vi "Main Page.vi"(8 "error in":errorcluster, 11 "Node Ptr":T1 format="%.0x") -> (0 "error out":errorcluster)   [LabVIEW 2026, in "SystemMonitor System Explorer.lvlib"]
uses:
  <vilib>/NI VeriStand/Custom Device API/Custom Device Item Ref.ctl
  <vilib>/NI VeriStand/Custom Device API/Get Item Property (U16).vi
  <vilib>/NI VeriStand/Custom Device API/Set Item Property (U16).vi
  SystemMonitor System Explorer.lvlib
  <vilib>/NI VeriStand/Custom Device API/Custom Device API.lvlib
  C:/Program Files/National Instruments/VeriStand 2026/NationalInstruments.VeriStand.Controls.dll
  Program Files/National Instruments/VeriStand 2026/NationalInstruments.VeriStand.Controls.dll
panel:
  in  "Timeout":u16 caption="Async Timeout (ms)"
  in  "PagePropertyEditor":refnum<k24>(container)
  out "Version":string
  in  "Browser":refnum<k7>(container)
  in  "General Header":cluster{"Section Name":string}={"Section Name"="General Custom Device Settings"}
  in  "Description":string
  in  "Name":string
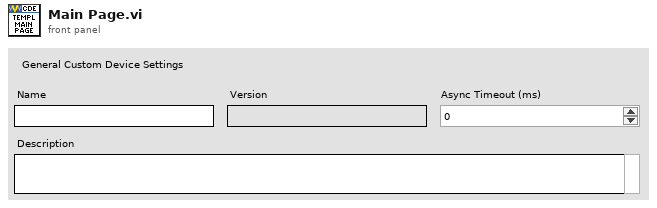
[diagram p1: front panel]
types:
  T1 = typedef "Custom Device API.lvlib/Custom Device Item Ref.ctl" = u64
  T2 = typedef "Custom Device API.lvlib/Custom Device Item Info.ctl" = cluster{"Name":string, "Is Channel":bool, "GUID":string, "Is Waveform":bool}
  T3 = typedef "Custom Device API.lvlib/Custom Device Commands.ctl" = enum16{"Default", "Item renamed", "Shutdown", "Dynamic button pressed"}
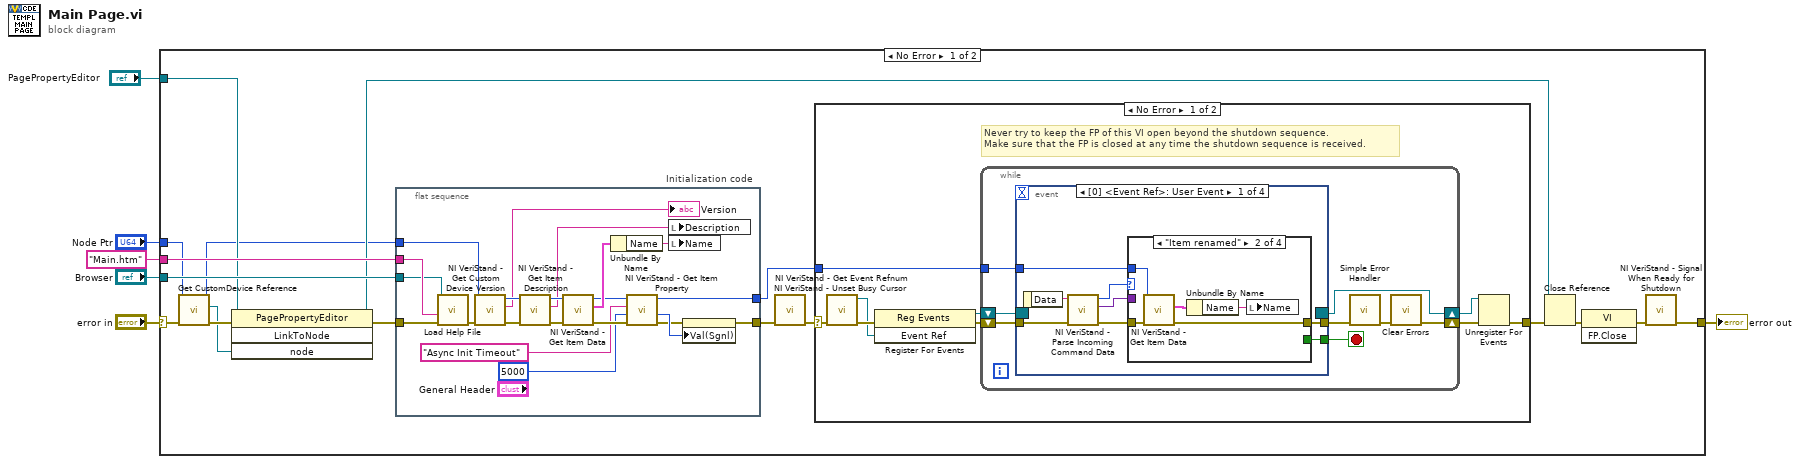
[diagram p0: block diagram]
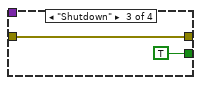
[diagram p3: hidden frame]
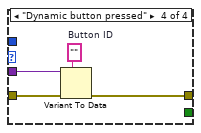
[diagram p4: hidden frame]
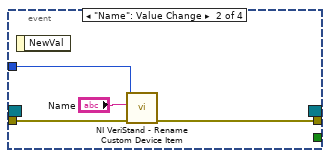
[diagram p5: hidden frame]
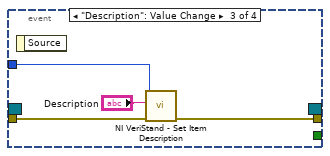
[diagram p6: hidden frame]
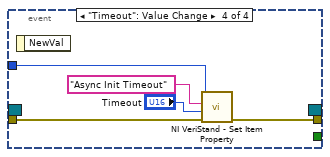
[diagram p7: hidden frame]
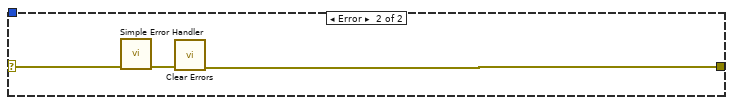
[diagram p8: hidden frame]
diagram:
  n1 = case shown="No Error" "error in" {
    selector: "error in" -> [w16 w98]
    tunnel: [w23 w98] -> w2
    tunnel: "Node Ptr" -> [w7 _]
    tunnel: "Browser" -> [w22 _]
    tunnel: "Main.htm" ("HTML File") -> [w21 _]
    tunnel: "PagePropertyEditor" -> [w9 _]
    frame No Error {
      n2 = call "Get CustomDevice Reference.vi"("error in"=w16, "Node Ptr"=w7) -> ("error out"=w12:errorcluster, "Custom Device"=w11:refnum<k24>, "Node Ptr"=w8:T1)  [unwired: 7 in]
      n3 = invoke class="PagePropertyEditor" method="LinkToNode"(reference=w9, error in=w12, "node"=w11) -> (reference out=w10:refnum<k24>, error out=w15:errorcluster)  [unwired: 1 in, 2 out]
      n4 = flat-sequence "Initialization code" {
        tunnel: w15 -> [w42]
        tunnel: w8 -> [w38]
        tunnel: [w24] -> w17
        tunnel: [w30] -> w18
        tunnel: w22 -> [w32]
        tunnel: w21 -> [w33]
        frame #0 {
          n5 = call "Load Help File.vi"("error in"=w42, "HTML File to Load"=w33, "Browser"=w32) -> ("error out"=w41:errorcluster)  [unwired: 8 in]
          n6 = call <vilib>:"NI VeriStand - Get Custom Device Version.vi"("error in (no error)"=w41, "Device Ref in"=w38) -> ("error out"=w43:errorcluster, "Value"=→"Version":string, "Device Ref out"=w37:T1)  [unwired: 7 in]
          n7 = call <vilib>:"NI VeriStand - Get Item Description.vi"("error in (no error)"=w43, "Item Ref in"=w37) -> ("error out"=w44:errorcluster, "Description"=w34:string, "Item Ref out"=w40:T1)  [unwired: 7 out]
          n8 = call <vilib>:"NI VeriStand - Get Item Data.vi"("error in (no error)"=w44, "Item Ref in"=w40) -> ("error out"=w29:errorcluster, "Item Info"=w39:T2, "Item Ref out"=w31:T1)  [unwired: 7 out]
          n9 = Unbundle By Name(w39) -> ("Name"=w35:string)
          n10 = call-poly <vilib>:"NI VeriStand - Get Item Property.vi"("error in (no error)"=w29, "Default Value"=u16 5000, "Property Name"="Async Init Timeout", "Item Ref in"=w31) -> ("error out"=w25:errorcluster, "Value"=w26:u16, "Item Ref out"=w30:T1)  [unwired: 4 in, 1 out]
          n11 = local write "Description"(w34) -> ()
          n12 = local write "Name"(w35) -> ()
          n13 = property on="Timeout" class="DigNum (strict)"(error in=w25, "Val(Sgnl)"=w26) -> (error out=w24:errorcluster)  [unwired: 1 in, 1 out]
        }
      }
      n14 = call <vilib>:"NI VeriStand - Unset Busy Cursor.vi"("error in (no error)"=w17) -> ("error out"=w19:errorcluster)  [unwired: 10 out]
      n15 = case shown="No Error" w19 {
        selector: w19 -> [w49 w97]
        tunnel: [w51 w95] -> w14
        tunnel: w18 -> [w45 _]
        frame No Error {
          # "Never try to keep the FP of this VI open beyond the shutdown sequence.\nMake sure that the FP is closed at any time the shutdown sequence is received."
          n16 = call <vilib>:"NI VeriStand - Get Event Refnum.vi"("error in (no error)"=w49) -> ("error out"=w53:errorcluster, "Event Ref"=w47:refnum<user-event>)  [unwired: 9 out]
          n17 = register-events(error in=w53, w47) -> (reference out=w46:refnum<event-registration>, error out=w50:errorcluster)  [unwired: 1 in]
          n18 = while {
            tunnel: w45 -> [w54]
            shift-right: [w58] -> w52
            shift-left: w50 -> [w61]
            shift-right: [w57] -> w48
            shift-left: w46 -> [w56]
            stop <- w55 stop-if-true
            n19 = event shown="[0] <Event Ref>: User Event" {
              selector: w56 -> [_ _ _ _]
              dyn-events: [_ _ _ _] -> w57
              timeout: _ -> [_ _ _ _]
              tunnel: w61 -> [w69 w85 w89 w94]
              tunnel: [w64 _ _ _] -> w55
              tunnel: [w67 w84 w88 w93] -> w60
              tunnel: w54 -> [w63 w83 w87 w91]
              event User Event {
                n20 = event-data() -> ("Data"=w66:string)  [unwired: 1 out]
                n21 = call <vilib>:"NI VeriStand - Parse Incoming Command Data.vi"("error in (no error)"=w69, "Incoming data"=w66) -> ("error out"=w68:errorcluster, "Outgoing data"=w62:variant, "Action"=w65:T3)  [unwired: 7 out]
                n22 = case shown="\"Item renamed\"" w65 {
                  tunnel: w68 -> [w70 w75 w77 w81]
                  tunnel: [_ _ TRUE _] -> w64
                  tunnel: [w70 w74 w77 w80] -> w67
                  tunnel: w63 -> [_ w73 _ _]
                  tunnel: w62 -> [_ _ _ w79]
                  frame "Default", Default {
                  }
                  frame "Item renamed" {
                    n23 = call <vilib>:"NI VeriStand - Get Item Data.vi"("error in (no error)"=w75, "Item Ref in"=w73) -> ("error out"=w74:errorcluster, "Item Info"=w72:T2)  [unwired: 8 out]
                    n24 = Unbundle By Name(w72) -> ("Name"=w71:string)
                    n25 = local write "Name"(w71) -> ()
                  }
                  frame "Shutdown" {
                  }
                  frame "Dynamic button pressed" {
                    w78 = ""  # Button ID
                    n26 = Variant To Data(error in=w81, type=w78, Variant=w79) -> (error out=w80:errorcluster)  [unwired: 1 out]
                  }
                }
              }
              event "Name": Value Change {
                n27 = event-data() -> ()  [unwired: 2 out]
                n28 = call <vilib>:"NI VeriStand - Rename Custom Device Item.vi"("error in (no error)"=w85, "New Name"="Name", "Item Ref in"=w83) -> ("error out"=w84:errorcluster)  [unwired: 1 in, 7 out]
              }
              event "Description": Value Change {
                n29 = event-data() -> ()  [unwired: 2 out]
                n30 = call <vilib>:"NI VeriStand - Set Item Description.vi"("error in (no error)"=w89, "Description"="Description", "Item Ref in"=w87) -> ("error out"=w88:errorcluster)  [unwired: 8 out]
              }
              event "Timeout": Value Change {
                n31 = event-data() -> ()  [unwired: 2 out]
                n32 = call-poly <vilib>:"NI VeriStand - Set Item Property.vi"("error in (no error)"=w94, "Value"="Timeout", "Property Name"="Async Init Timeout", "Item Ref in"=w91) -> ("error out"=w93:errorcluster)  [unwired: 5 in, 2 out]
              }
            }
            n33 = call <vilib>:"Simple Error Handler.vi"("error in (no error)"=w60) -> ("error out"=w59:errorcluster)  [unwired: 1 in, 7 out]
            n34 = call <vilib>:"Clear Errors.vi"("error in (no error)"=w59) -> ("error out"=w58:errorcluster)  [unwired: 1 in, 5 out]
          }
          n35 = Unregister For Events(event registration refnum=w48, error in=w52) -> (error out=w51:errorcluster)
        }
        frame Error {
          n36 = call <vilib>:"Simple Error Handler.vi"("error in (no error)"=w97) -> ("error out"=w96:errorcluster)  [unwired: 1 in, 7 out]
          n37 = call <vilib>:"Clear Errors.vi"("error in (no error)"=w96) -> ("error out"=w95:errorcluster)  [unwired: 1 in, 5 out]
        }
      }
      n38 = Close Reference(reference=w10, error in (no error)=w14) -> (error out=w13:errorcluster)
      n39 = invoke class="VI" method="FP.Close"(error in=w13) -> (error out=w20:errorcluster)  [unwired: 2 in, 2 out]
      n40 = call <vilib>:"NI VeriStand - Signal When Ready for Shutdown.vi"("error in (no error)"=w20) -> ("error out"=w23:errorcluster)  [unwired: 10 out]
    }
    frame Error {
    }
  }
  "error out" <- w2
